vi "i2cTests.vi"() -> ()   [LabVIEW 2016]
uses:
  VIs/uPythonX/uPythonX.xctl
panel:
  in  "uPythonX 3":T1(xcontrol)={"VISA Refnum in"="ASRL23::INSTR", "Python Code"="#SLAVE\nfrom machine import I2CSlaveMem\n\nmem = bytearray(16)\nfor i in range(16):\n     mem[i] = i\n\ni2c_slave = I2CSlaveMem('Y', 55, mem)\n\n\n#MASTER \nimport machine,pyb\n\ni2c_master = machine.I2C(scl=pyb.Pin('X1'), sda=pyb.Pin('X2'), freq=5000)\n\ni2c_master.scan()\n\nfred = i2c_master.readfrom_mem(55, 8, 3)\ni2c_master.writeto_mem(55, 2, b'\\x10')"}
  in  "uPythonX 2":T1(xcontrol)={"VISA Refnum in"="ASRL23::INSTR", "Python Code"="from machine import I2C\n\n\ni2c = I2C('Y', freq=10000)\ni2c.scan()\n\n\nmem = bytearray(16)\nfor i in range(16):\n     mem[i] = i\n"}
  in  "Python Code":string="from machine import I2CSlaveMem\n\nmem = bytearray(16)\nfor i in range(16):\n     mem[i] = i\n\ni2c_slave = I2CSlaveMem(port = 2, 4, mem)       \n\n\n\nfrom machine import I2C\n\ni2c = I2C('Y', freq=100000)\ni2c.scan()\n\nfred = i2c.readfrom_mem(42, 8, 3)\ni2c.writeto_mem(42,2,'1')"
  in  "uPythonX":T1(xcontrol)={"VISA Refnum in"="ASRL32::INSTR", "Python Code"="from machine import I2CSlaveMem\n\nmem = bytearray(16)\nfor i in range(16):\n     mem[i] = i+2\n     \nmem\n\ni2c_slave = I2CSlaveMem('Y', 32, mem)\nmem\n\nmem"}
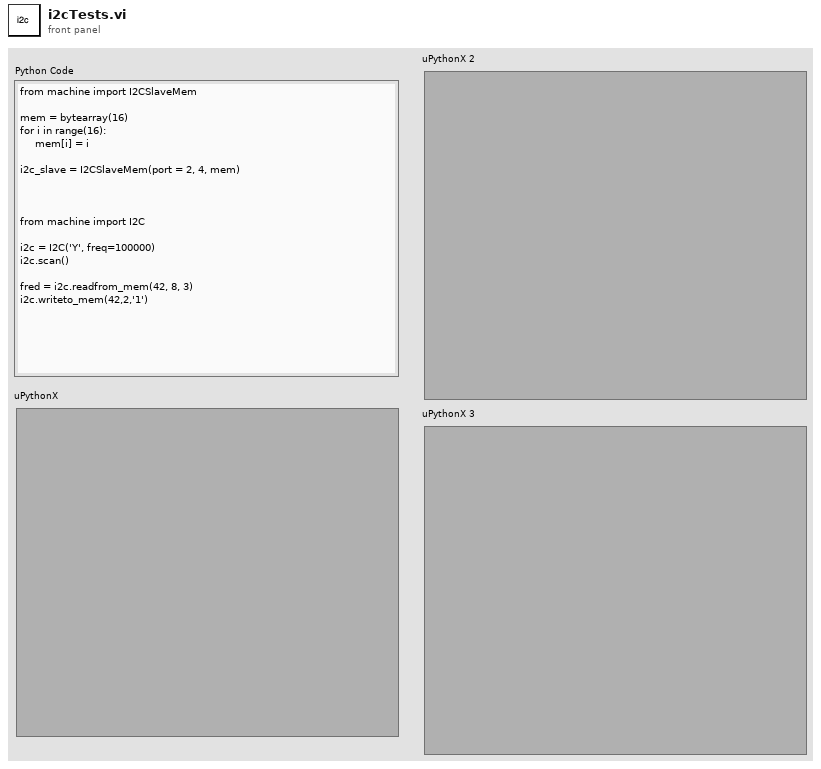
[diagram p1: front panel]
types:
  T1 = cluster{"VISA Refnum in":refnum<visa-resource-name>, "Python Code":string}
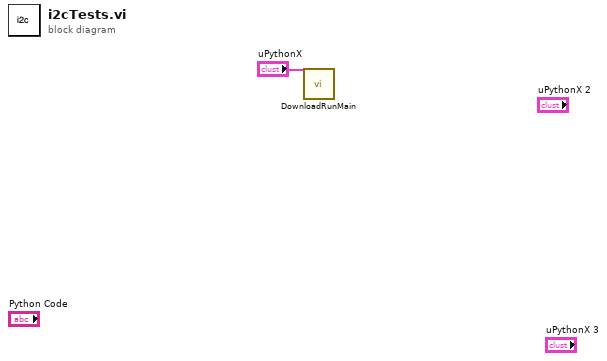
[diagram p0: block diagram]
diagram:
  n1 = call "DownloadRunMain.vi"("uPythonX"="uPythonX") -> ()  [unwired: 8 in, 3 out]
